vi "osie na grafie.vi"(11 "axis info":T1) -> (3 "graph 2":cluster{i32[], i32[]}[](graph))   [LabVIEW 2015]
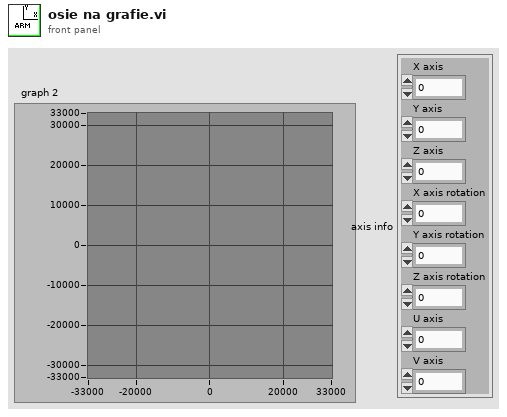
[diagram p1: front panel]
types:
  T1 = cluster{"X axis":i32, "Y axis":i32, "Z axis":i32, "X axis rotation":i32, "Y axis rotation":i32, "Z axis rotation":i32, "U axis":i32, "V axis":i32}
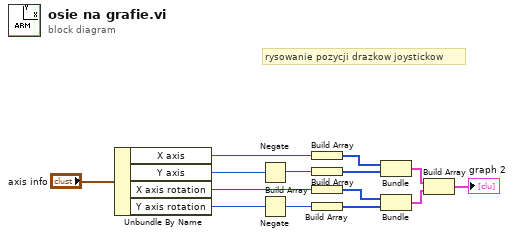
[diagram p0: block diagram]
diagram:
  # "rysowanie pozycji drazkow joystickow"
  n1 = Unbundle By Name("axis info") -> ("X axis"=w4:i32, "Y axis"=w3:i32, "X axis rotation"=w2:i32, "Y axis rotation"=w1:i32)
  n2 = Negate(x=w3) -> (-x=w9:i32)
  n3 = Negate(x=w1) -> (-x=w6:i32)
  n4 = Build Array(w4) -> (w11:i32[])
  n5 = Build Array(w9) -> (w10:i32[])
  n6 = Build Array(w2) -> (w8:i32[])
  n7 = Build Array(w6) -> (w7:i32[])
  n8 = Bundle(w11, w10) -> (w13:cluster{i32[], i32[]})  [unwired: 1 in]
  n9 = Bundle(w8, w7) -> (w12:cluster{i32[], i32[]})  [unwired: 1 in]
  n10 = Build Array(w13, w12) -> (→"graph 2":cluster{i32[], i32[]}[])
